vi "LucaContinuousDisplay.vi"() -> ()   [LabVIEW 2009]
panel:
  out "last":i32
  out "first":u32
  in  "Stop":bool
  out "Intensity Graph":u16[][](graph)
  in  "Acquisition Timeout":i32=1000
  in  "Bin Size":i32=1
  in  "Exposure Time":sgl=0.3 format="%.2f"
  in  "EMCCD Gain":i32=200
  in  "Camera Index":i32=1
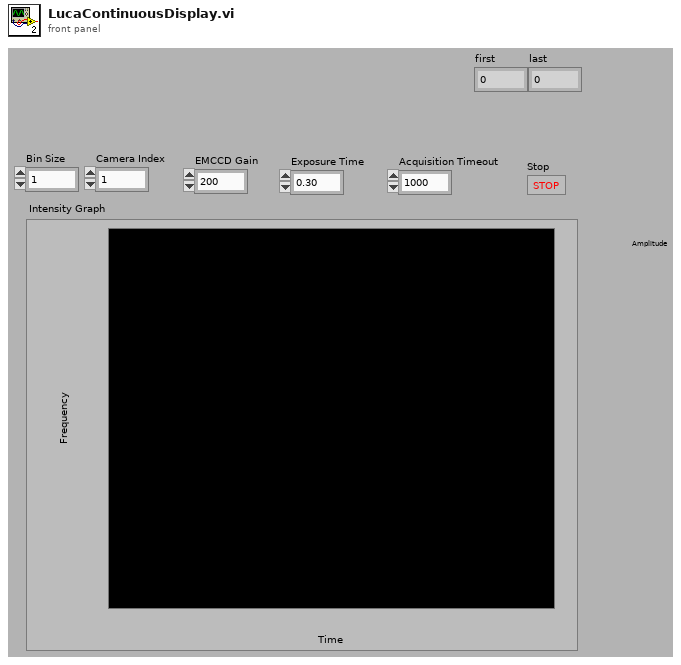
[diagram p1: front panel]
types:
  T1 = cluster{"left":i32, "right":i32, "top":i32, "bottom":i32}
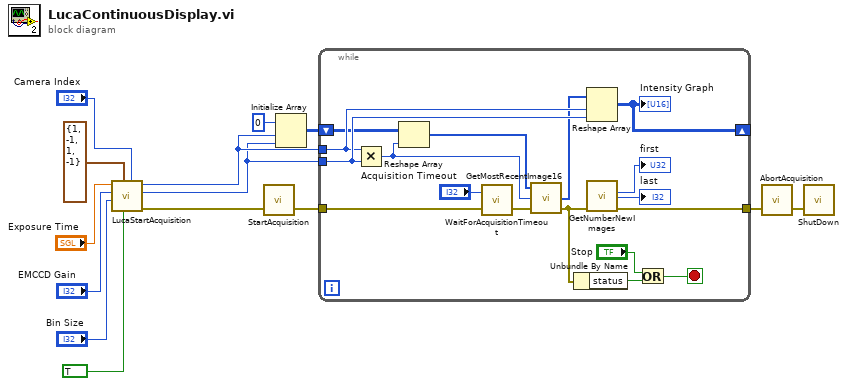
[diagram p0: block diagram]
diagram:
  n1 = call "LucaStartAcquisition.vi"("Camera Index"="Camera Index", "Continuous"=TRUE, "input cluster"=T1 {"left"=1, "right"=-1, "top"=1, "bottom"=-1}, "Bin Size"="Bin Size", "EMCCD Gain"="EMCCD Gain", "Exposure Time"="Exposure Time") -> ("error out"=w11:errorcluster, "VSize"=w3:i32, "HSize"=w4:i32)  [unwired: 3 in]
  n2 = call <userlib>:"StartAcquisition.vi"("error in (no error)"=w11) -> ("error out"=w2:errorcluster)  [unwired: 1 in, 1 out]
  n3 = Initialize Array(i16 0, w4, w3) -> (w14:i16[][])
  n4 = while {
    tunnel: w4 -> [w27]
    tunnel: w3 -> [w28]
    tunnel: w2 -> [w29]
    shift-right: [w20] -> _
    shift-left: w14 -> [w26]
    tunnel: [w17] -> w5
    stop <- w30 stop-if-true
    n5 = Multiply(x=w27, y=w28) -> (x*y=w23:i32)
    n6 = Reshape Array(w26, w23) -> (w22:u16[])
    n7 = call <userlib>:"WaitForAcquisitionTimeout.vi"("error in (no error)"=w29, "iTimeOutMs"="Acquisition Timeout") -> ("error out"=w25:errorcluster)  [unwired: 1 out]
    n8 = call <userlib>:"GetMostRecentImage16.vi"("error in (no error)"=w25, "size"=w23, "array"=w22) -> ("error out"=w18:errorcluster, "array"=w24:u16[])  [unwired: 1 out]
    n9 = Unbundle By Name(w18) -> ("status"=w31:bool)
    n10 = Reshape Array(w24, w27, w28) -> (w20:u16[][])
    "Intensity Graph" <- w20
    n11 = call <userlib>:"GetNumberNewImages.vi"("error in (no error)"=w18) -> ("error out"=w17:errorcluster, "last"=→"last":i32, "first"=→"first":u32)  [unwired: 3 in, 1 out]
    n12 = Or(x="Stop", y=w31) -> (x .or. y?=w30:bool)
  }
  n13 = call <userlib>:"AbortAcquisition.vi"("error in (no error)"=w5) -> ("error out"=w12:errorcluster)  [unwired: 1 in, 1 out]
  n14 = call <userlib>:"ShutDown.vi"("error in (no error)"=w12) -> ()  [unwired: 1 in, 2 out]
